vi "Read Section - I32.vi"(4 "Default":i32, 6 "Create file if not found? (T)":bool=TRUE, 8 "error in (no error)":errorcluster, 9 "key":string, 10 "section":string, 11 "Path":path) -> (0 "error out":errorcluster, 3 "value":i32)   [LabVIEW 2019, in "TSC File IO.lvlib"]
doc: "This VI will read a section/key configuration file and return:\n<b>I32 (integer)</b>\n\nInputs:\n-Path [path] - a path to the file\n-section [string] - the section string in the configuration file\n-key [string] - the key to be read in the configuration file\n-error in\n\nOutputs:\n-value [I32] - the output data read\n-error out\n\n<b>Code Developed By:</b>\nDaniel Coons\nTechnology Service Corporation\n1983 S Liberty Drive\nBloomington, IN 47403\nwww.tsc.com\\atcs"
uses:
  TSC File IO.lvlib
  <vilib>/Utility/config.llb/Read Key (I32).vi
  <vilib>/Utility/config.llb/NI_LVConfig.lvlib
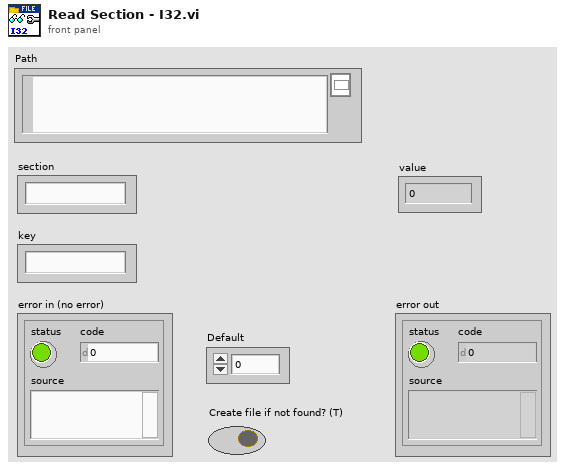
[diagram p1: front panel]
types:
  T1 = typedef "NI_LVConfig.lvlib/Config Data RefNum.ctl" = refnum<k1>
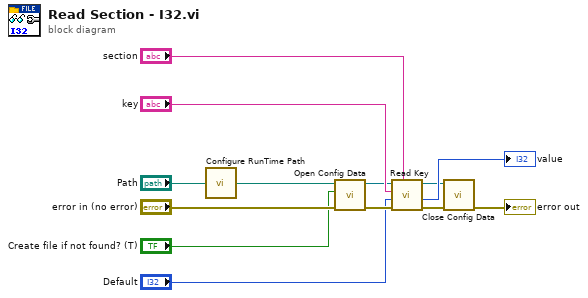
[diagram p0: block diagram]
diagram:
  n1 = call "Configure RunTime Path.vi"("Input Path"="Path") -> ("Updated Path"=w3:path)
  n2 = call <vilib>:"Open Config Data.vi"("error in (no error)"="error in (no error)", "create file if necessary (T)"="Create file if not found? (T)", "configuration file path"=w3) -> ("error out"=w4:errorcluster, "refnum"=w5:T1)  [unwired: 6 in, 1 out]
  n3 = call-poly <vilib>:"Read Key.vi"("section"="section", "error in (no error)"=w4, "default value"="Default", "key"="key", "refnum"=w5) -> ("error out"=w6:errorcluster, "value"=→"value":i32, "refnum out"=w7:T1)  [unwired: 3 in, 1 out]
  n4 = call <vilib>:"Close Config Data.vi"("error in (no error)"=w6, "refnum"=w7) -> ("error out"=→"error out":errorcluster)  [unwired: 8 in, 1 out]
